vi "Send Write Desired Temperature.vi"(7 "Message Priority (Normal)":T1=enum."Normal", 8 "error in (no error)":errorcluster, 10 "Desired Temperature":dbl=75.0, 11 "Message Enqueuer":refnum<class "Message Enqueuer.lvclass">) -> (0 "error out":errorcluster)   [LabVIEW 2018, in "Cooler.lvlib" / "Write Desired Temperature Msg.lvclass"]
doc: "This VI sends the message to an actor."
uses:
  Write Desired Temperature Msg.lvclass
  <vilib>/ActorFramework/Message Enqueuer/Message Enqueuer.lvclass
  <vilib>/ActorFramework/Message Enqueuer/Message Priority.ctl
  e:/builds/penguin/labview/branches/2018/dev/dist/vi.lib/ActorFramework/Message/Message.lvclass
  Write Desired Temperature Msg.lvclass/Write Desired Temperature Msg.ctl
  <vilib>/ActorFramework/Message Enqueuer/Message Enqueuer.lvclass/Message Enqueuer.ctl
  <vilib>/ActorFramework/Message Priority Queue/Priority Enqueue.vi
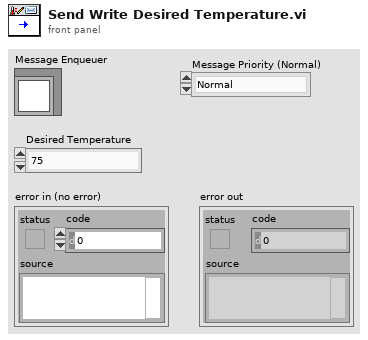
[diagram p1: front panel]
types:
  T1 = typedef "Actor Framework.lvlib/Message Enqueuer.lvclass/Message Priority.ctl" = enum16{"Low", "Normal", "High"}
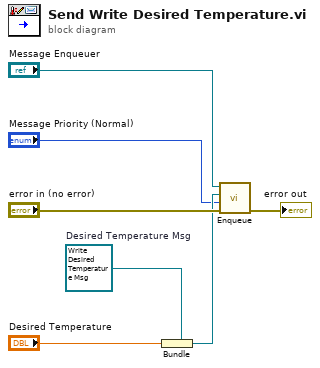
[diagram p0: block diagram]
diagram:
  w4 = refnum<class "Write Desired Temperature Msg.lvclass"> refnum  # Desired Temperature Msg
  n1 = Bundle(cluster=w4, "Desired Temperature") -> (w3:refnum<class "Write Desired Temperature Msg.lvclass">)
  n2 = call <vilib>:"Enqueue.vi"("error in (no error)"="error in (no error)", "Message Priority (Normal)"="Message Priority (Normal)", "Message"=w3, "Message Enqueuer in"="Message Enqueuer") -> ("error out"=→"error out":errorcluster)  [unwired: 6 in, 1 out]
